vi "oa_Check Vector Reference is Empty (1 Channel).vi"(0 "magnitudes [RMS] in":T1(array[cluster]) {"magnitude" format="%.2f"; "time/rev/rpm" format="%.2f"}, 2 "reset? (F)":bool, 5 "phases [phase lag] in":cluster{"time/rev/rpm":dbl[], "phase":dbl[]}[](array[cluster]) {"phase" format="%.2f"; "time/rev/rpm" format="%.2f"}, 11 "error in (no error)":errorcluster) -> (4 "magnitudes [RMS] out":T1(array[cluster]) {"magnitude" format="%.2f"; "time/rev/rpm" format="%.2f"}, 6 "phases [phase lag] out":cluster{"time/rev/rpm":dbl[], "phase":dbl[]}[](array[cluster]) {"phase" format="%.2f"; "time/rev/rpm" format="%.2f"}, 8 "empty?":bool, 15 "error out":errorcluster)   [LabVIEW 2017, in "SoundVib_RefDataProcess.lvlib"]
uses:
  <vilib>/addons/Sound and Vibration/Order Analysis/Referece Data Processing/SoundVib_RefDataProcess.lvlib
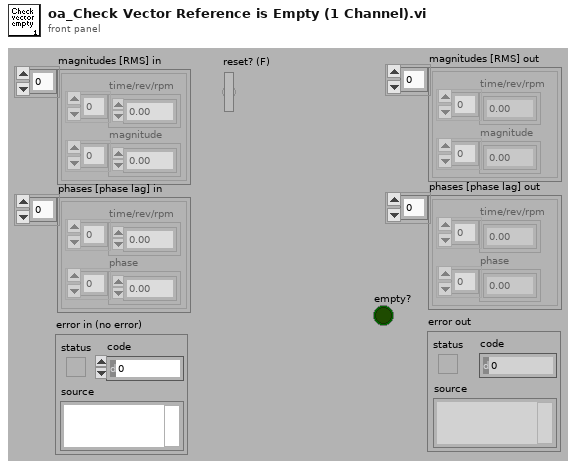
[diagram p1: front panel]
types:
  T1 = cluster{"time/rev/rpm":dbl[], "magnitude":dbl[]}[]
  T2 = cluster{"is warning? (False)":bool, "error code (0)":i32, "error message (\"\")":string}
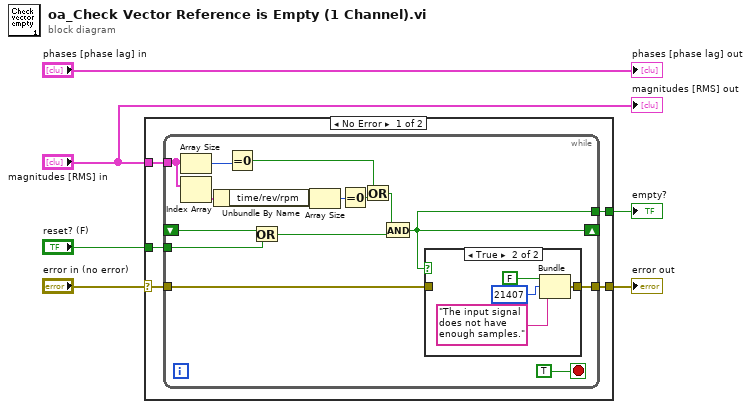
[diagram p0: block diagram]
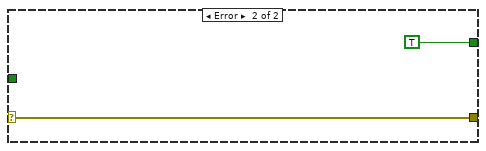
[diagram p3: hidden frame]
diagram:
  n1 = case shown="No Error" "error in (no error)" {
    selector: "error in (no error)" -> [w10 w32]
    tunnel: "magnitudes [RMS] in" -> [w11 _]
    tunnel: [w8 TRUE] -> w4
    tunnel: [w9 w32] -> w2
    tunnel: "reset? (F)" -> [w7 _]
    frame No Error {
      n2 = while {
        tunnel: w11 -> [w25]
        tunnel: w10 -> [w19]
        tunnel: [w18] -> w9
        shift-right: [w12] -> _
        shift-left: _ -> [w14]
        tunnel: [w12] -> w8
        tunnel: w7 -> [w15]
        stop <- TRUE stop-if-true
        n3 = Array Size(array=w25) -> (size(s)=w26:i32)
        n4 = Index Array(array=w25) -> (element=w24:cluster{"time/rev/rpm":dbl[], "magnitude":dbl[]})  [unwired: 1 in]
        n5 = Unbundle By Name(w24) -> ("time/rev/rpm"=w23:dbl[])
        n6 = Equal To 0?(x=w26) -> (x = 0?=w20:bool)
        n7 = Or(x=w14, y=w15) -> (x .or. y?=w13:bool)
        n8 = Array Size(array=w23) -> (size(s)=w21:i32)
        n9 = Equal To 0?(x=w21) -> (x = 0?=w22:bool)
        n10 = Or(x=w20, y=w22) -> (x .or. y?=w16:bool)
        n11 = And(x=w16, y=w13) -> (x .and. y?=w12:bool)
        n12 = case shown="True" w12 {
          tunnel: w19 -> [w27 _]
          tunnel: [w27 w28] -> w18
          frame False {
          }
          frame True {
            n13 = Bundle("is warning? (False)"=FALSE, "error code (0)"=21407, "error message (\"\")"="The input signal does not have enough samples." ("error message (\"\")")) -> (w28:T2)  [unwired: 1 in]
          }
        }
      }
    }
    frame Error {
    }
  }
  "empty?" <- w4
  "error out" <- w2
  "magnitudes [RMS] out" <- "magnitudes [RMS] in"
  "phases [phase lag] out" <- "phases [phase lag] in"
